vi "qam.vi"() -> ()   [LabVIEW 2026]
panel:
  out "Constellation IQ":cluster{dbl[], dbl[]}(graph)
  in  "Nsymbols":dbl
  out "Bandwidth":dbl
  out "Spectre FFT":dbl[](graph)
  out "Signal QAM":dbl[](graph)
  in  "alpha":dbl
  in  "fc":dbl
  in  "Fe":dbl
  in  "Rs":dbl
  in  "M":dbl
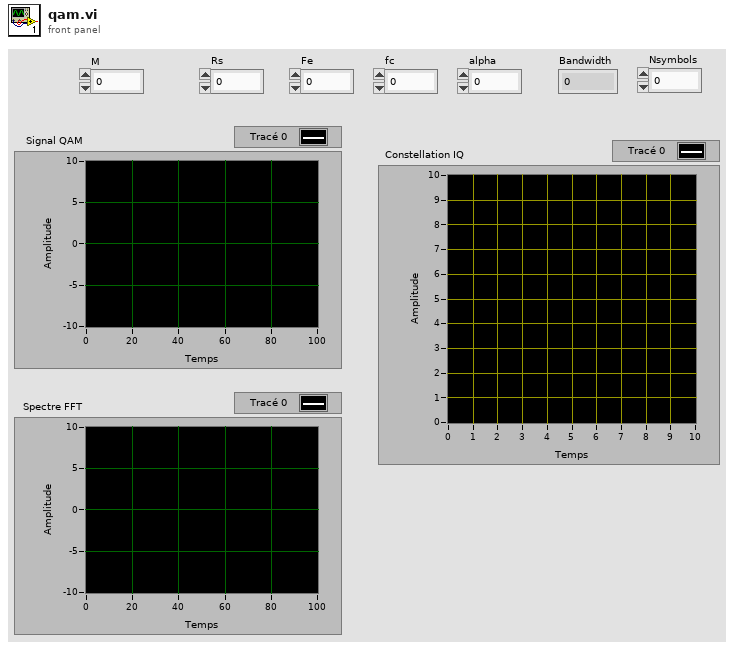
[diagram p1: front panel]
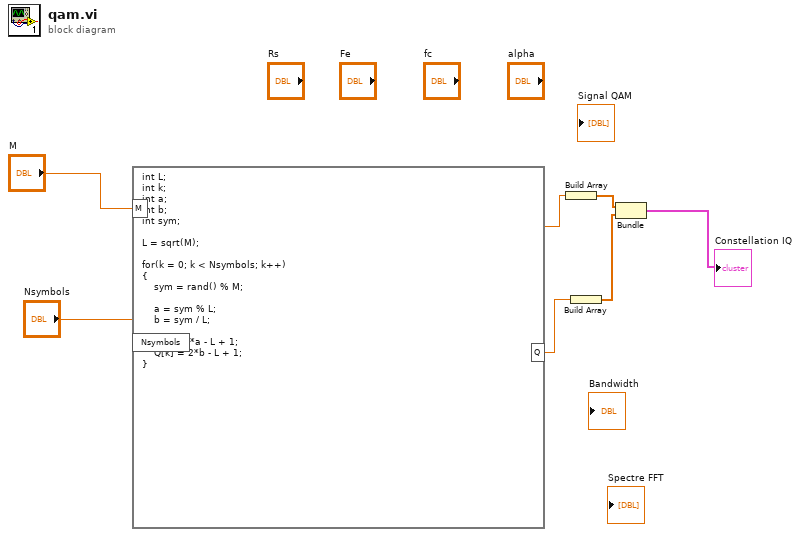
[diagram p0: block diagram]
diagram:
  n1 = formula code="int L;\nint k;\nint a;\nint b;\nint sym;\n\nL = sqrt(M);\n\nfor(k = 0; k < Nsymbols; k++)\n{\n    sym = rand() % M;\n\n    a = sym % L;\n    b = sym / L;\n\n    I[k] = 2*a - L + 1;\n    Q[k] = 2*b - L + 1;\n}"("M"="M", "Nsymbols"="Nsymbols") -> (w1:dbl, "Q"=w5:dbl)
  n2 = Build Array(w1) -> (w4:dbl[])
  n3 = Build Array(w5) -> (w3:dbl[])
  n4 = Bundle(w4, w3) -> (→"Constellation IQ":cluster{dbl[], dbl[]})  [unwired: 1 in]
